vi "Value to U32 string.vi"(1 "Value":u32) -> (0 "U32 str (Little Endian)":string)   [LabVIEW 2015]
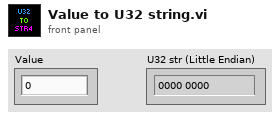
[diagram p1: front panel]
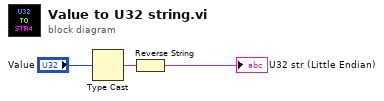
[diagram p0: block diagram]
diagram:
  n1 = Type Cast(x="Value") -> (*(type *) &x=w3:string)  [unwired: 1 in]
  n2 = Reverse String(1:w3) -> (0:→"U32 str (Little Endian)":string)
